vi "rtout_getTriggerConfig.vi"(0 "connection ID":refnum<k5>, 1 "axis":i32, 5 "error in":errorcluster) -> (13 "polarity":i32, 14 "connection ID":refnum<k5>, 15 "axis_out":i32, 16 "higher":i32, 17 "lower":i32, 18 "epsilon":i32, 19 "error out":errorcluster)   [LabVIEW 2016, in "AMC_VIs.lvlib"]
doc: "Get the real time output trigger config"
uses:
  AMC_VIs.lvlib
panel:
  out "params_cluster":cluster{"axis":i32}
  in  "Params_cluster":cluster{"integer":i32}
  in  "results_cluster":T1
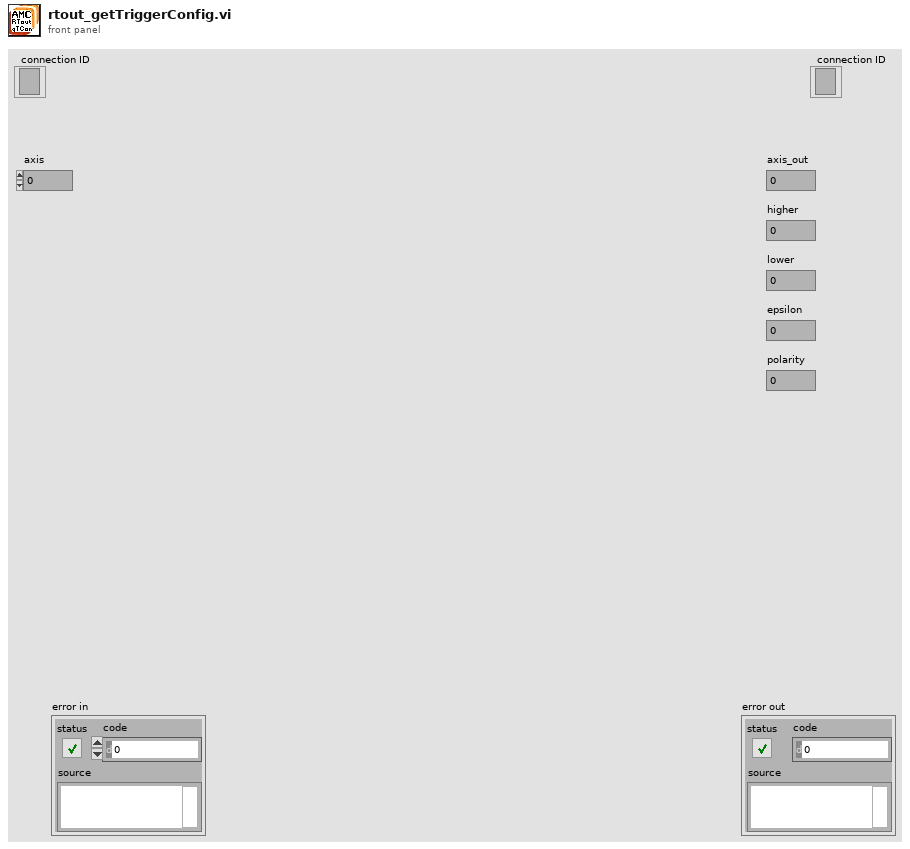
[diagram p1: front panel]
types:
  T1 = cluster{"errNo":i32, "higher":i32, "lower":i32, "epsilon":i32, "polarity":i32}
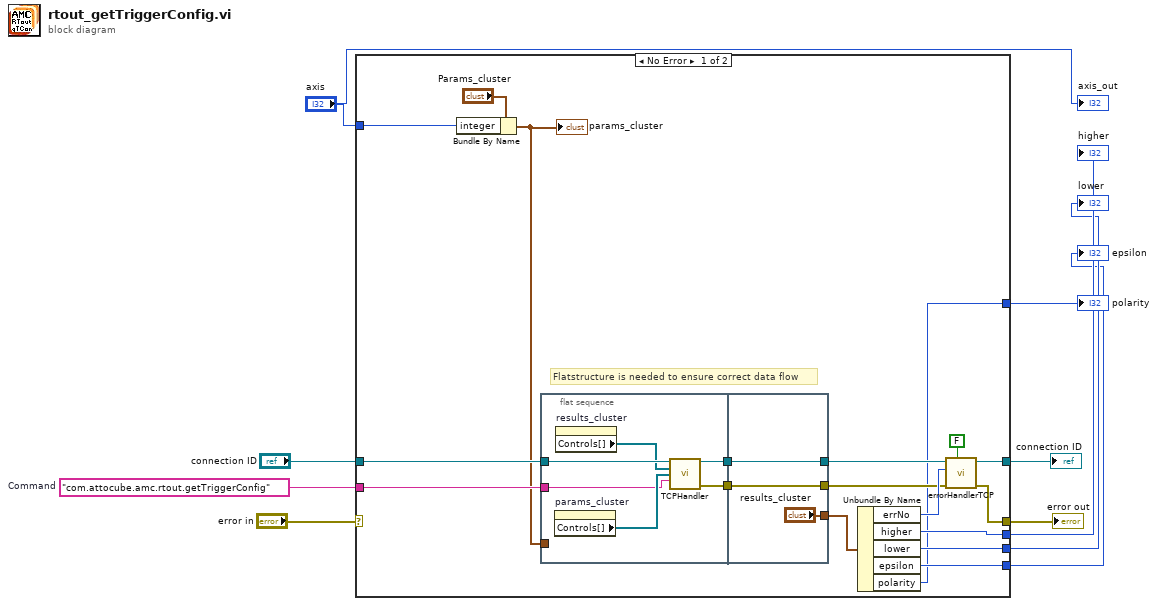
[diagram p0: block diagram]
diagram:
  w6 = "com.attocube.amc.rtout.getTriggerConfig"  # Command
  n1 = case shown="No Error" "error in" {
    selector: "error in" -> [_ w39]
    tunnel: [w26 w39] -> w10
    tunnel: [w28 w38] -> w9
    tunnel: "connection ID" -> [w25 w38]
    tunnel: w6 -> [w19 _]
    tunnel: "axis" -> [w15 _]
    tunnel: [w14 _] -> w4
    tunnel: [w13 _] -> w3
    tunnel: [w12 _] -> w2
    tunnel: [w11 _] -> w1
    frame No Error {
      # "Flatstructure is needed to ensure correct data flow"
      n2 = Bundle By Name(cluster="Params_cluster", "integer"=w15) -> (w16:cluster{"integer":i32})
      "params_cluster" <- w16
      n3 = flat-sequence {
        tunnel: [w33] -> w21
        tunnel: w25 -> [w34]
        tunnel: w19 -> [w30]
        tunnel: [w29] -> w17
        tunnel: w16 -> [_]
        tunnel: ["results_cluster"] -> w22
        tunnel: [w37] -> w24
        tunnel: w21 -> [w37]
        tunnel: [w35] -> w18
        tunnel: w17 -> [w35]
        frame #0 {
          n4 = property on="params_cluster" class="Clust (strict)"() -> ("Controls[]"=w31:refnum<vi>[])  [unwired: 2 in, 2 out]
          n5 = property on="results_cluster" class="Clust (strict)"() -> ("Controls[]"=w32:refnum<vi>[])  [unwired: 2 in, 2 out]
          n6 = call "TCPHandler.vi"("connection ID"=w34, "results_cluster"=w32, "params_cluster"=w31, "method"=w30) -> ("connection ID"=w33:refnum<k5>, "error"=w29:errorcluster)  [unwired: 8 in, 2 out]
        }
        frame #1 {
        }
      }
      n7 = Unbundle By Name(w22) -> ("errNo"=w23:i32, "higher"=w14:i32, "lower"=w13:i32, "epsilon"=w12:i32, "polarity"=w11:i32)
      n8 = call "errorHandlerTCP.vi"("show popup"=FALSE, "error in"=w18, "error number"=w23, "connection ID"=w24) -> ("error out"=w26:errorcluster, "connection ID"=w28:refnum<k5>)  [unwired: 6 in]
    }
    frame Error {
    }
  }
  "error out" <- w10
  "connection ID" <- w9
  "higher" <- w4
  "lower" <- w3
  "epsilon" <- w2
  "polarity" <- w1
  "axis_out" <- "axis"
